vi "saveDataToFile.vi"(1 "data":string, 2 "fileRefnum":refnum<file>) -> ()   [LabVIEW 2010]
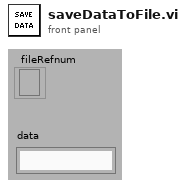
[diagram p1: front panel]
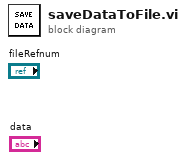
[diagram p0: block diagram]
diagram:
